vi "Table_Recurse Through Children.vi"(8 "error in":errorcluster, 9 "TreeBrowser":refnum<k24>, 10 "Children":refnum<k24>[](array[refnum]), 11 ".NET Refnum in":refnum<k24>) -> (0 "error out":errorcluster, 2 "Children":refnum<k24>[](array[refnum]))   [LabVIEW 2012, in "TableSupportLib.lvlib"]
uses:
  TableSupportLib.lvlib
  NationalInstruments.VeriStand.SystemDefinitionAPI
  NationalInstruments.VeriStand.SystemStorageUI
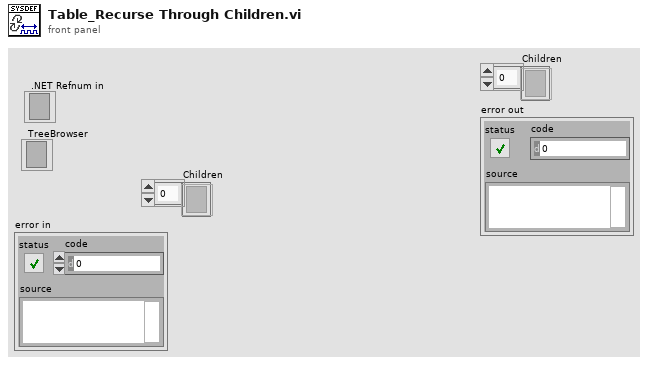
[diagram p1: front panel]
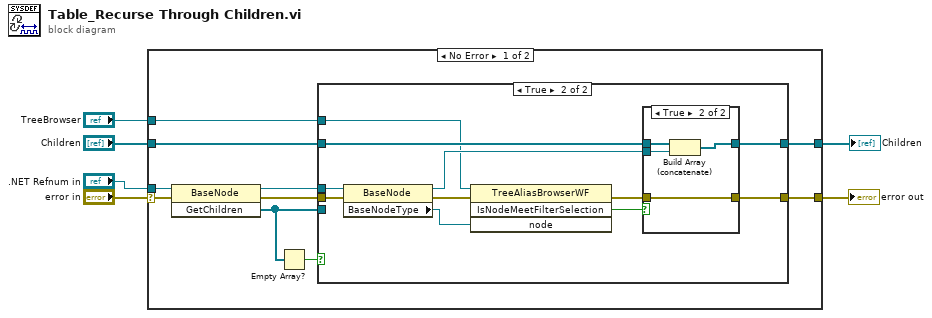
[diagram p0: block diagram]
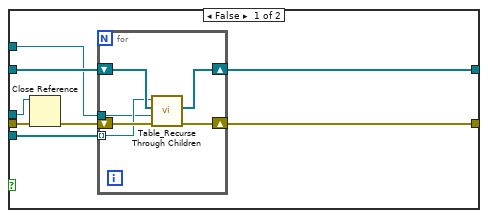
[diagram p2: hidden frame]
diagram:
  n1 = case shown="No Error" "error in" {
    selector: "error in" -> [w10 w49]
    tunnel: ".NET Refnum in" -> [w9 _]
    tunnel: "Children" -> [w16 w48]
    tunnel: [w15 w48] -> w4
    tunnel: [w8 w49] -> w3
    tunnel: "TreeBrowser" -> [w7 _]
    frame No Error {
      n2 = invoke class="BaseNode" method="GetChildren"(reference=w9, error in=w10) -> (reference out=w13:refnum<k24>, error out=w12:errorcluster, "GetChildren"=w14:refnum<k24>[])  [unwired: 1 in]
      n3 = Empty Array?(array=w14) -> (empty?=w11:bool)
      n4 = case shown="True" w11 {
        tunnel: w14 -> [w24 _]
        tunnel: w16 -> [w23 w41]
        tunnel: w13 -> [w18 w39]
        tunnel: [w22 w40] -> w15
        tunnel: w12 -> [w20 w37]
        tunnel: [w21 w33] -> w8
        tunnel: w7 -> [w17 w31]
        frame False {
          n5 = Close Reference(reference=w18, error in (no error)=w20) -> (error out=w19:errorcluster)
          n6 = for {
            tunnel: w24 -> [w27] mode=indexing
            shift-right: [w29] -> w22
            shift-left: w23 -> [w30]
            shift-right: [w26] -> w21
            shift-left: w19 -> [w28]
            tunnel: w17 -> [w25]
            n7 = call "Table_Recurse Through Children.vi"("error in"=w28, "TreeBrowser"=w25, "Children"=w30, ".NET Refnum in"=w27) -> ("error out"=w26:errorcluster, "Children"=w29:refnum<k24>[])  [unwired: 6 in]
          }
        }
        frame True {
          n8 = property class="BaseNode"(reference=w39, error in=w37) -> (reference out=w34:refnum<k24>, error out=w36:errorcluster, "BaseNodeType"=w38:refnum<k24>)
          n9 = invoke class="TreeAliasBrowserWF" method="IsNodeMeetFilterSelection"(reference=w31, error in=w36, "node"=w38) -> (error out=w32:errorcluster, "IsNodeMeetFilterSelection"=w35:bool)  [unwired: 1 in, 2 out]
          n10 = case shown="True" w35 {
            tunnel: w41 -> [w43 w47]
            tunnel: [w43 w46] -> w40
            tunnel: w34 -> [_ w45]
            tunnel: [w42 w44] -> w33
            tunnel: w32 -> [w42 w44]
            frame False {
            }
            frame True {
              n11 = Build Array (concatenate)(w47, w45) -> (w46:refnum<k24>[])
            }
          }
        }
      }
    }
    frame Error {
    }
  }
  "Children" <- w4
  "error out" <- w3
